vi "Test_output_mixing_2.vi"() -> ()   [LabVIEW 2013]
uses:
  <vilib>/measure/maspectr.llb/Power Spectrum and PSD Export Mode.ctl
  <vilib>/measure/maspectr.llb/FFT Power Spectrum and PSD for 1 Chan.vi
  <vilib>/measure/NI_MAPro.lvlib
panel:
  out "output array 2":i16[](array[numeric])
  out "data out 3":i16[](graph)
  out "size(s) 2":i32
  out "power spectrum":cluster{"f0":dbl, "df":dbl, "magnitude":dbl[]}(graph)
  out "data out 2":dbl[][](graph)
  out "size(s)":i32
  out "s? t:f":i32
  out "data out":i16[](graph)
  out "# elements":i32
  out "output array":i16[](array[numeric])
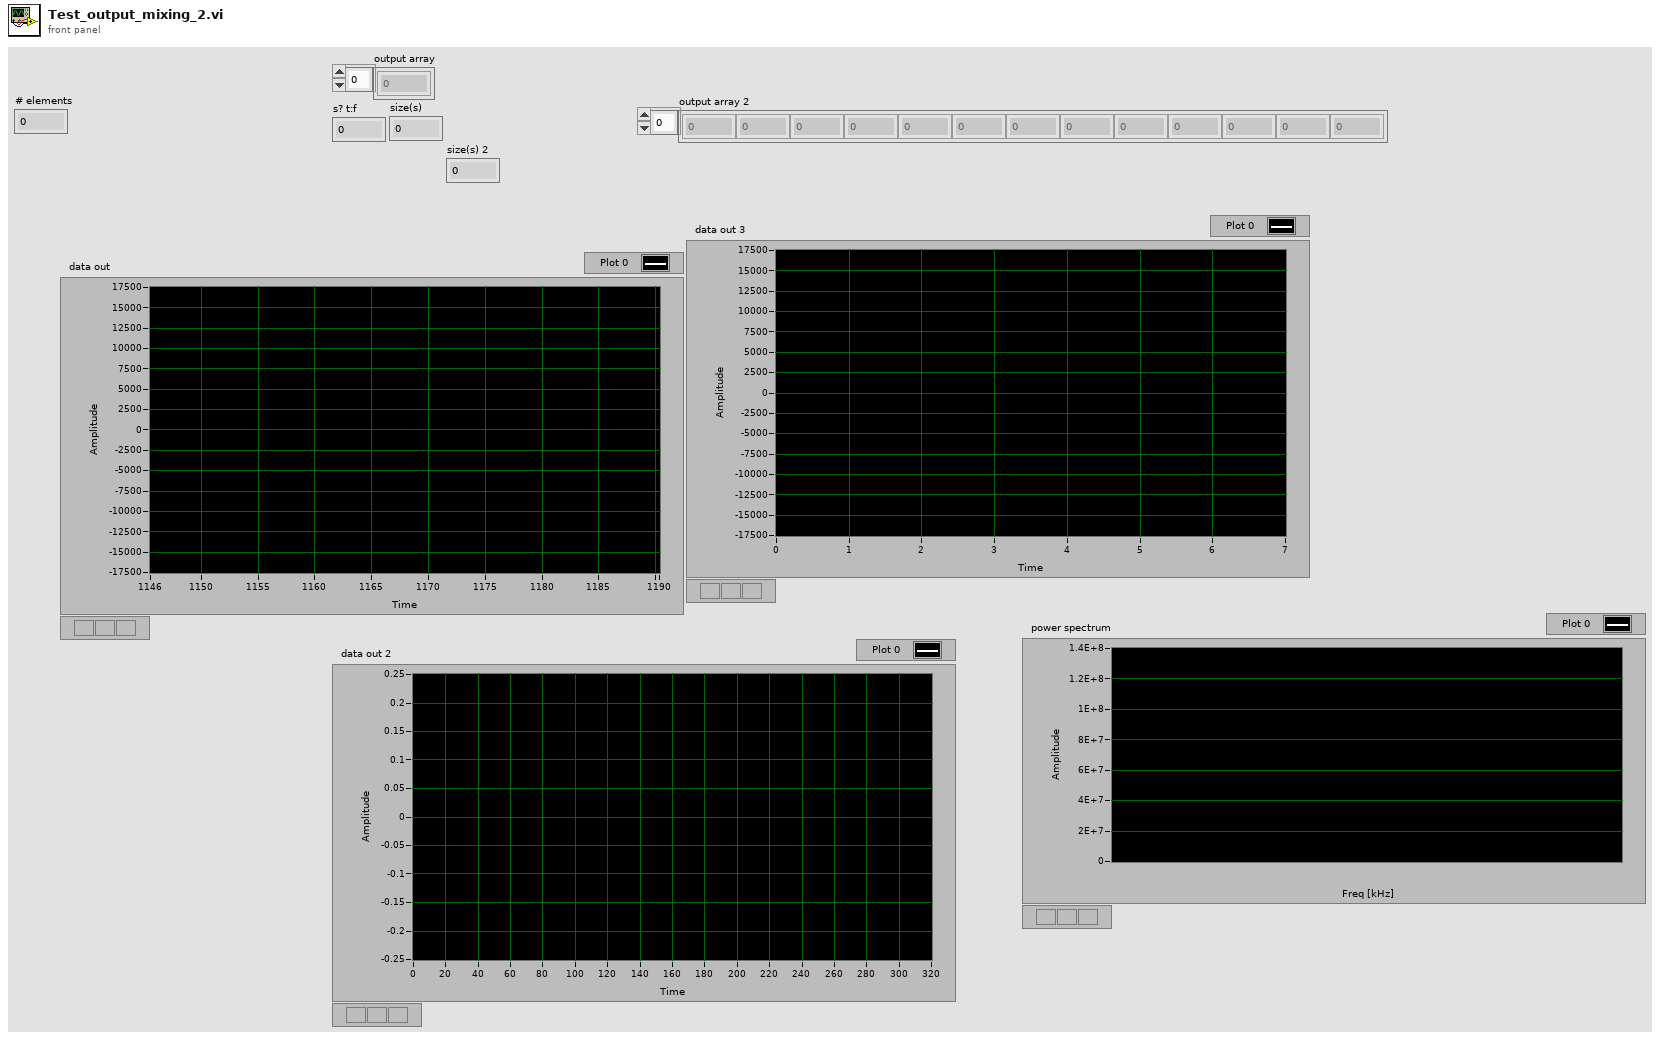
[diagram p1: front panel]
types:
  T1 = typedef "NI_MAPro.lvlib/Power Spectrum and PSD Export Mode.ctl" = u16
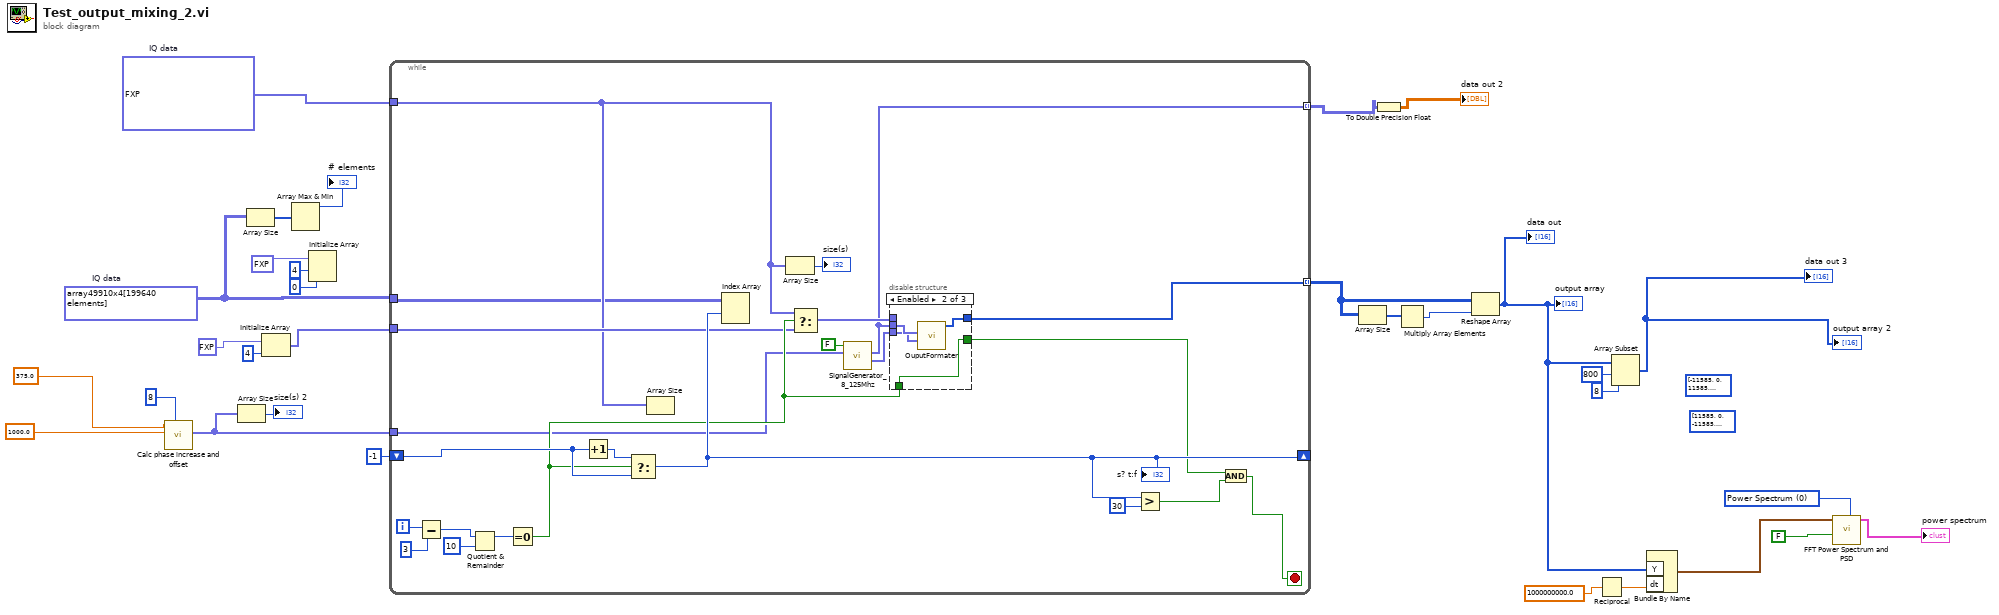
[diagram p0: block diagram]
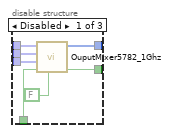
[diagram p2: hidden frame]
diagram:
  (unwired) i16[] [-11585, 0, 11585, -16384, 11585, 0, -11585, 16384] ("output array 2")
  (unwired) i16[] [11585, 0, -11585, -16384, -11585, 0, 11585, 16384] ("output array 2")
  w12 = T1 0 items=["Power Spectrum", "Power Spectral Density"] ("export mode")
  w16 = fxp<+/-,16,14>[] [200.0, 0.0, 0.0, 0.0]  # IQ data
  w24 = fxp<+/-,16,14>[][] array49910x4[199640 elements]  # IQ data
  n1 = call "Calc phase increase and offset.vi"("# of DDS"=8, "fclk (MHz)"=1000.0 ("fclk (800MHz)"), "f_generated (MHz)"=375.0) -> ("Phase out"=w6:fxp<+,64,64>[])  [unwired: 6 in, 2 out]
  n2 = Array Size(array=w6) -> (size(s)=→"size(s) 2":i32)
  n3 = Array Size(array=w24) -> (size(s)=w26:i32[])
  n4 = Initialize Array(fxp<+/-,16,14> 0.0 ("Q out"), 4 ("dimension size")) -> (w21:fxp<+/-,16,14>[])
  n5 = Array Max & Min(array=w26) -> (max value=→"# elements":i32)  [unwired: 3 out]
  n6 = Initialize Array(fxp<+,7,8> 250.0 ("Q out"), 4 ("dimension size"), 0 ("dimension size")) -> ()  [unwired: 1 out]
  n7 = while {
    tunnel: w24 -> [w34]
    shift-right: [w50] -> _
    shift-left: -1 -> [w51]
    tunnel: [w32] -> w13 mode=indexing
    tunnel: w6 -> [w40]
    tunnel: w21 -> [w39]
    tunnel: w16 -> [w35]
    tunnel: [w33] -> w14 mode=indexing
    i -> [w49]
    stop <- w45 stop-if-true
    n8 = Subtract(x=w49, y=3) -> (x-y=w47:i32)
    n9 = Quotient & Remainder(x=w47, y=10) -> (x-y*floor(x/y)=w53:i32)  [unwired: 1 out]
    n10 = Equal To 0?(x=w53) -> (x = 0?=w44:bool)
    n11 = Increment(x=w51) -> (x+1=w52:i32)
    n12 = Select(t=w52, s=w44, f=w51) -> (s? t:f=w50:i32)
    "s? t:f" <- w50
    n13 = Array Size(array=w35) -> ()  [unwired: 1 out]
    n14 = Index Array(array=w34, index (row)=w50) -> ()  [unwired: 1 in, 1 out]
    n15 = Array Size(array=w35) -> (size(s)=→"size(s)":i32)
    n16 = Select(t=w35, s=w44, f=w39) -> (s? t:f=w42:fxp<+/-,16,14>[])
    n17 = call "SignalGenerator_8_125Mhz.vi"("Phase"=w40, "reset"=FALSE) -> ("Sine out"=w38:fxp<+/-,16,0>[], "Cosine out"=w33:fxp<+/-,16,0>[])  [unwired: 8 in]
    n18 = disable-structure shown="Enabled" {
      disable-tunnel: w44 -> [w61 w63 w66]
      disable-tunnel: [w60 w63 w66] -> w43
      disable-tunnel: w42 -> [w59 _ _]
      disable-tunnel: w38 -> [w57 w62 _]
      disable-tunnel: w33 -> [w56 w65 w67]
      disable-tunnel: [w55 w64 w67] -> w32
      frame Disabled {
        n19 = call "OuputMixer5782_1Ghz.vi"("reset"=FALSE, "valid in"=w61, "Sine in"=w57, "Cosine in"=w56, "Data in"=w59) -> ("valid out"=w60:bool, "test"=w55:i16[])  [unwired: 5 in]
      }
      frame Enabled {
        n20 = call "OuputFormater.vi"("Sine in"=w62, "Cosine in"=w65) -> ("test"=w64:i16[])  [unwired: 9 in]
      }
      frame Disabled {
      }
    }
    n21 = Greater?(x=w50, y=30) -> (0:w46:bool)
    n22 = And(x=w43, y=w46) -> (x .and. y?=w45:bool)
  }
  n23 = Array Size(array=w13) -> (size(s)=w28:i32[])
  n24 = To Double Precision Float(number=w14) -> (double precision float=→"data out 2":dbl[][])
  n25 = Multiply Array Elements(1:w28) -> (0:w27:i32)
  n26 = Reshape Array(w13, w27) -> (w4:i16[])
  "output array" <- w4
  "data out" <- w4
  n27 = Reciprocal(x=1000000000.0 ("dt")) -> (1/x=w8:dbl)
  n28 = Array Subset(array=w4, index=800, length=8) -> (→"output array 2" →"data out 3":i16[])
  n29 = Bundle By Name("Y"=w4, "dt"=w8) -> (w11:waveform(i16))  [unwired: 1 in]
  n30 = call-poly <vilib>:"FFT Power Spectrum and PSD.vi"("export mode"=w12, "dB On (F)"=FALSE, "time signal"=w11) -> ("Power Spectrum / PSD"=→"power spectrum":cluster{"f0":dbl, "df":dbl, "magnitude":dbl[]})  [unwired: 5 in, 3 out]
